vi "p29_1_eul2rot.vi"() -> ()   [LabVIEW 2013]
uses:
  <vilib>/Analysis/coordinate.llb/Euler Rotation Order.ctl
  <vilib>/Analysis/NI_AALPro.lvlib
panel:
  out "R":picture
  out "gamma":cluster{"phi":dbl, "theta":dbl, "psi":dbl}={"phi"=0.10000000000000009, "theta"=0.2, "psi"=0.2999999999999998}
  out "gamma (euler angles)":cluster{"phi":dbl, "theta":dbl, "psi":dbl}={"phi"=0.10000000000000009, "theta"=0.2, "psi"=0.2999999999999998}
  out "R 2":picture
  out "R":picture
  out "gamma (euler angles)":cluster{"phi":dbl, "theta":dbl, "psi":dbl}={"phi"=0.10000000000000009, "theta"=0.2, "psi"=0.2999999999999998}
  out "transformation matrix":picture
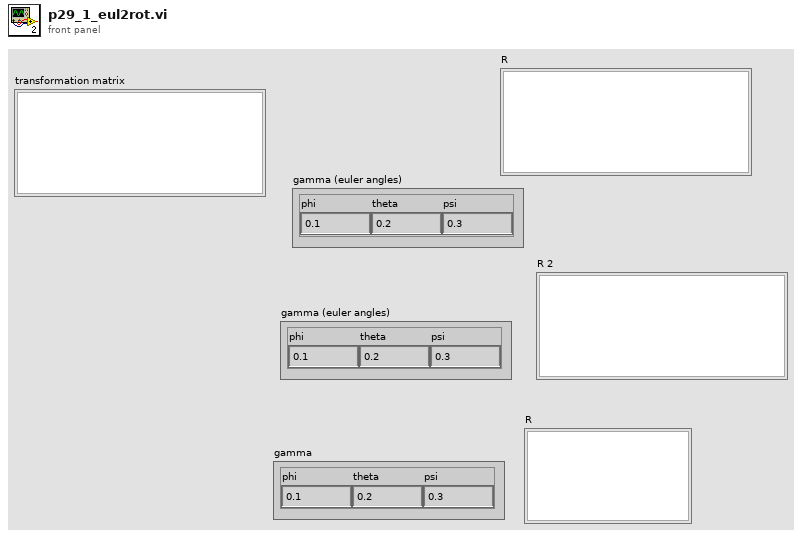
[diagram p1: front panel]
types:
  T1 = typedef "NI_AALPro.lvlib/Euler Rotation Order.ctl" = u16
  T2 = typedef "NI_Matrix.lvlib/RealMatrix.ctl" = dbl[][]
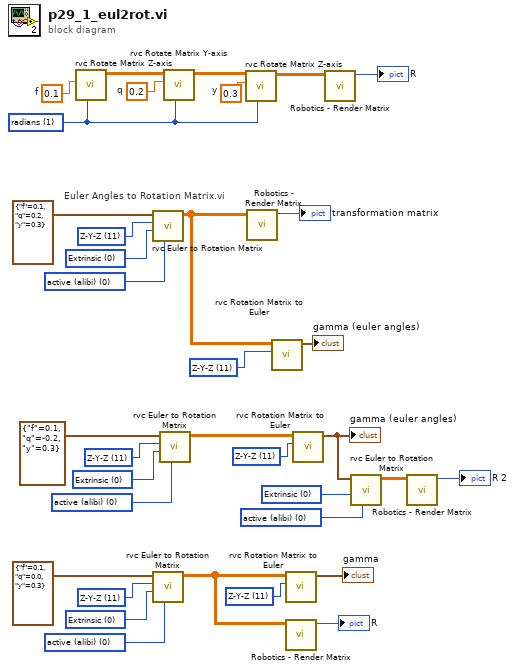
[diagram p0: block diagram]
diagram:
  w7 = T1 11 items=["X-Y-Z", "X-Z-Y", "Y-X-Z", "Y-Z-X", "Z-X-Y", "Z-Y-X", "X-Y-X", "X-Z-X", "Y-X-Y", "Y-Z-Y", "Z-X-Z", "Z-Y-Z"] ("rotation order")
  w3 = u16 0 items=["active (alibi)", "passive (alias)"] ("type of transformation")
  w5 = T1 11 items=["X-Y-Z", "X-Z-Y", "Y-X-Z", "Y-Z-X", "Z-X-Y", "Z-Y-X", "X-Y-X", "X-Z-X", "Y-X-Y", "Y-Z-Y", "Z-X-Z", "Z-Y-Z"] ("rotation order")
  w4 = u16 0 items=["Extrinsic", "Intrinsic"] ("type of rotations")
  w11 = T1 11 items=["X-Y-Z", "X-Z-Y", "Y-X-Z", "Y-Z-X", "Z-X-Y", "Z-Y-X", "X-Y-X", "X-Z-X", "Y-X-Y", "Y-Z-Y", "Z-X-Z", "Z-Y-Z"] ("rotation order")
  w15 = u16 0 items=["active (alibi)", "passive (alias)"] ("type of transformation")
  w13 = T1 11 items=["X-Y-Z", "X-Z-Y", "Y-X-Z", "Y-Z-X", "Z-X-Y", "Z-Y-X", "X-Y-X", "X-Z-X", "Y-X-Y", "Y-Z-Y", "Z-X-Z", "Z-Y-Z"] ("rotation order")
  w14 = u16 0 items=["Extrinsic", "Intrinsic"] ("type of rotations")
  w21 = u16 0 items=["active (alibi)", "passive (alias)"] ("type of transformation")
  w20 = u16 0 items=["Extrinsic", "Intrinsic"] ("type of rotations")
  w19 = T1 11 items=["X-Y-Z", "X-Z-Y", "Y-X-Z", "Y-Z-X", "Z-X-Y", "Z-Y-X", "X-Y-X", "X-Z-X", "Y-X-Y", "Y-Z-Y", "Z-X-Z", "Z-Y-Z"] ("rotation order")
  w23 = u16 1 items=["degree", "radians"] ("angle unit")
  w27 = 0.3  # y
  w30 = 0.2  # q
  w28 = 0.1  # f
  w31 = u16 0 items=["active (alibi)", "passive (alias)"] ("type of transformation")
  w33 = T1 11 items=["X-Y-Z", "X-Z-Y", "Y-X-Z", "Y-Z-X", "Z-X-Y", "Z-Y-X", "X-Y-X", "X-Z-X", "Y-X-Y", "Y-Z-Y", "Z-X-Z", "Z-Y-Z"] ("rotation order")
  w32 = u16 0 items=["Extrinsic", "Intrinsic"] ("type of rotations")
  # "Euler Angles to Rotation Matrix.vi"
  n1 = call "rvc Rotate Matrix Z-axis.vi"("angle unit"=w23, "angle"=w28) -> ("rotation matrix"=w26:T2)  [unwired: 9 in]
  n2 = call "rvc Euler to Rotation Matrix.vi"("type of transformation"=w31, "type of rotations"=w32, "rotation order"=w33, "euler angles"=cluster{"f":dbl, "q":dbl, "y":dbl} {"f"=0.1, "q"=0.2, "y"=0.3} ("angles")) -> ("rotation matrix"=w22:T2)  [unwired: 6 in, 1 out]
  n3 = call "rvc Euler to Rotation Matrix.vi"("type of transformation"=w3, "type of rotations"=w4, "rotation order"=w5, "euler angles"=cluster{"f":dbl, "q":dbl, "y":dbl} {"f"=0.1, "q"=0.0, "y"=0.3} ("angles")) -> ("rotation matrix"=w1:T2)  [unwired: 6 in, 1 out]
  n4 = call "rvc Euler to Rotation Matrix.vi"("type of transformation"=w15, "type of rotations"=w14, "rotation order"=w13, "euler angles"=cluster{"f":dbl, "q":dbl, "y":dbl} {"f"=0.1, "q"=-0.2, "y"=0.3} ("angles")) -> ("rotation matrix"=w10:T2)  [unwired: 6 in, 1 out]
  n5 = call "rvc Rotate Matrix Y-axis.vi"("angle unit"=w23, "angle"=w30, "rotation matrix in"=w26) -> ("rotation matrix"=w25:T2)  [unwired: 8 in]
  n6 = call "rvc Rotate Matrix Z-axis.vi"("angle unit"=w23, "angle"=w27, "rotation matrix in"=w25) -> ("rotation matrix"=w24:T2)  [unwired: 8 in]
  n7 = call "Robotics - Render Matrix.vi"("A"=w22) -> ("picture out"=→"transformation matrix":picture)  [unwired: 10 in]
  n8 = call "rvc Rotation Matrix to Euler.vi"("rotation order"=w19, "rotation matrix"=w22) -> ("euler angles"=→"gamma (euler angles)":cluster{"phi":dbl, "theta":dbl, "psi":dbl})  [unwired: 8 in, 1 out]
  n9 = call "rvc Rotation Matrix to Euler.vi"("rotation order"=w7, "rotation matrix"=w1) -> ("euler angles"=→"gamma":cluster{"phi":dbl, "theta":dbl, "psi":dbl})  [unwired: 8 in, 1 out]
  n10 = call "Robotics - Render Matrix.vi"("A"=w1) -> ("picture out"=→"R":picture)  [unwired: 10 in]
  n11 = call "rvc Rotation Matrix to Euler.vi"("rotation order"=w11, "rotation matrix"=w10) -> ("euler angles"=w9:cluster{"phi":dbl, "theta":dbl, "psi":dbl})  [unwired: 8 in, 1 out]
  "gamma (euler angles)" <- w9
  n12 = call "Robotics - Render Matrix.vi"("A"=w24) -> ("picture out"=→"R":picture)  [unwired: 10 in]
  n13 = call "rvc Euler to Rotation Matrix.vi"("type of transformation"=w21, "type of rotations"=w20, "euler angles"=w9) -> ("rotation matrix"=w17:T2)  [unwired: 7 in, 1 out]
  n14 = call "Robotics - Render Matrix.vi"("A"=w17) -> ("picture out"=→"R 2":picture)  [unwired: 10 in]
